vi "while_v0_v8.vi"() -> ()   [LabVIEW 2009]
panel:
  in  "Latime":i64(knob)=109 scale=0.0..220.0
  in  "Temporizare intre doua puncte afisate (ms)":dbl(slide)=4.313099041533546 scale=0.0..50.0
  out "Waveform Chart":i64(graph)
  in  "stop":bool
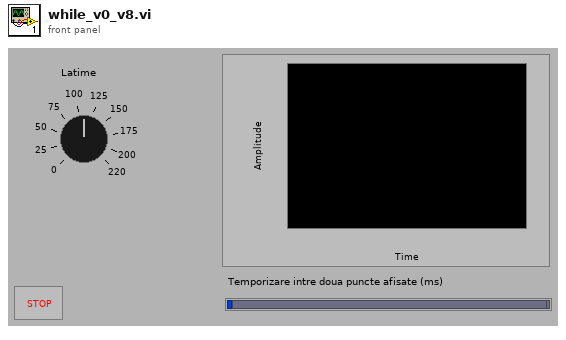
[diagram p1: front panel]
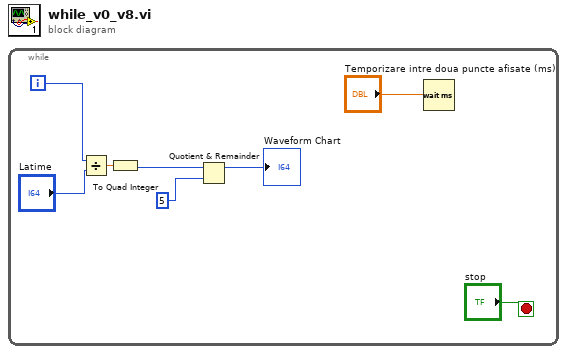
[diagram p0: block diagram]
diagram:
  n1 = while {
    i -> [w3]
    stop <- "stop" stop-if-true
    n2 = Divide(x=w3, y="Latime") -> (x/y=w4:dbl)
    n3 = To Quad Integer(1:w4) -> (0:w1:i64)
    n4 = Quotient & Remainder(x=w1, y=5) -> (x-y*floor(x/y)=→"Waveform Chart":i64)  [unwired: 1 out]
    n5 = Wait (ms)(milliseconds to wait="Temporizare intre doua puncte afisate (ms)") -> ()  [unwired: 1 out]
  }
